vi "RGBtoGray.vi"() -> ()   [LabVIEW 2019]
uses:
  <vilib>/vision/NI_Vision_Development_Module.lvlib
  RGB_To_Gray DLL Project/Project RGBToGray VI/RGBToGray.dll
panel:
  out "Gray Image Built In function":T1(plugin-control)
  out "Gray Image":T1(plugin-control)
  out "Execution Time in seconds (in DLL)":dbl
  out "Original Image":T1(plugin-control)
  in  "File Path":path
  out "Elapsed Time Labview Built in VI in ms":u32
  out "Elapsed Time For Our C DLL in ms":u32
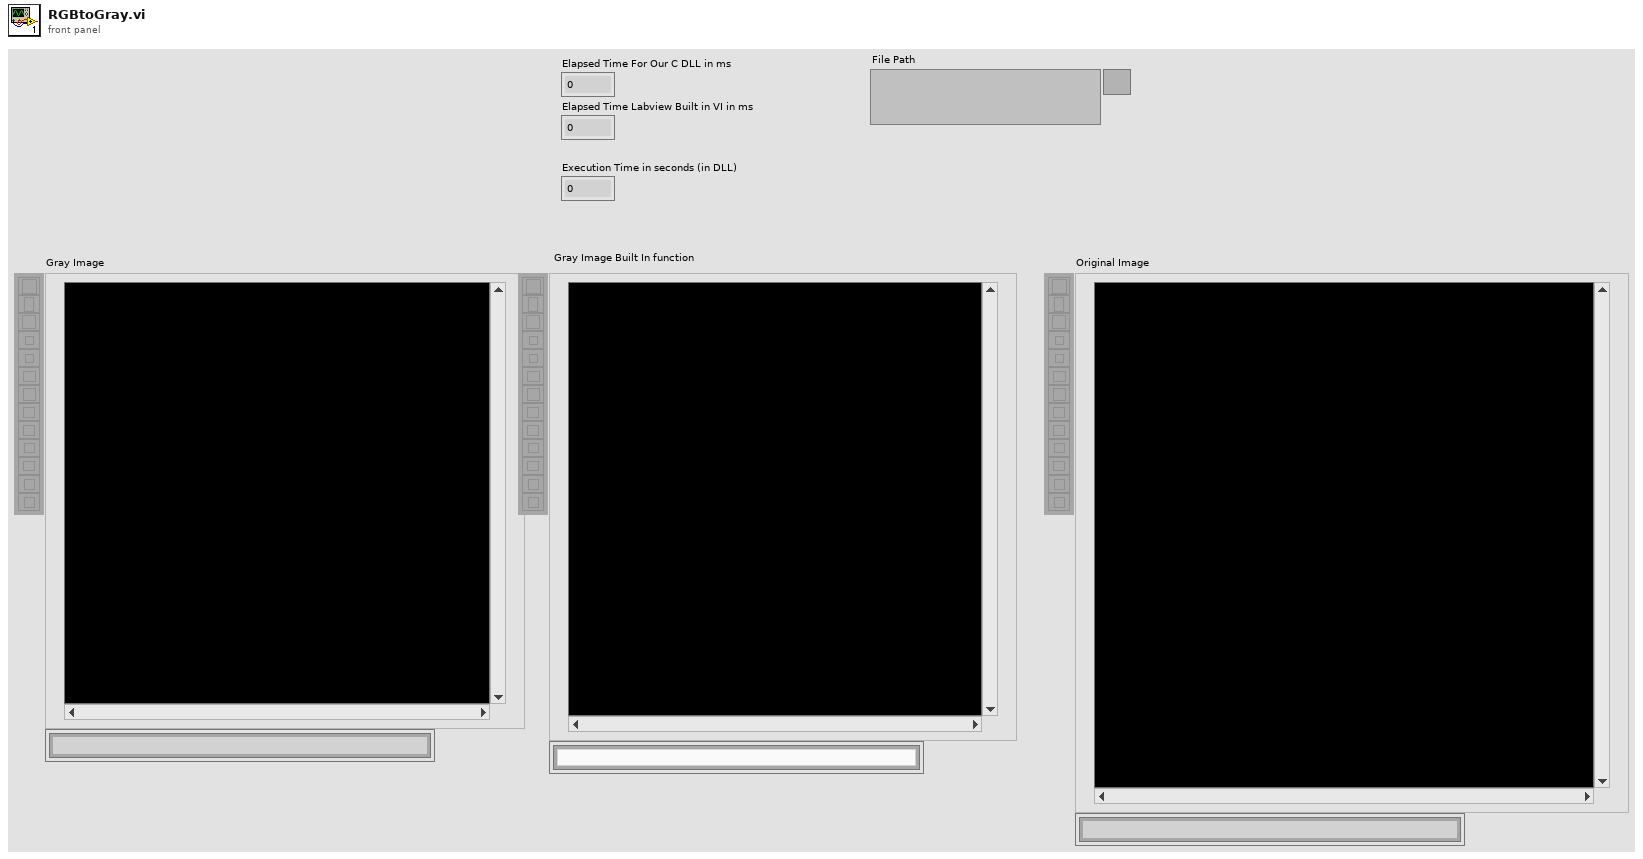
[diagram p1: front panel]
types:
  T1 = typedef "IMAQ Image.ctl" = refnum<image>
  T2 = enum32{"Map Pixel Pointer", "Unmap Pixel Pointer", "Get Pixels Infos"}
  T3 = typedef "Image Type" = u32
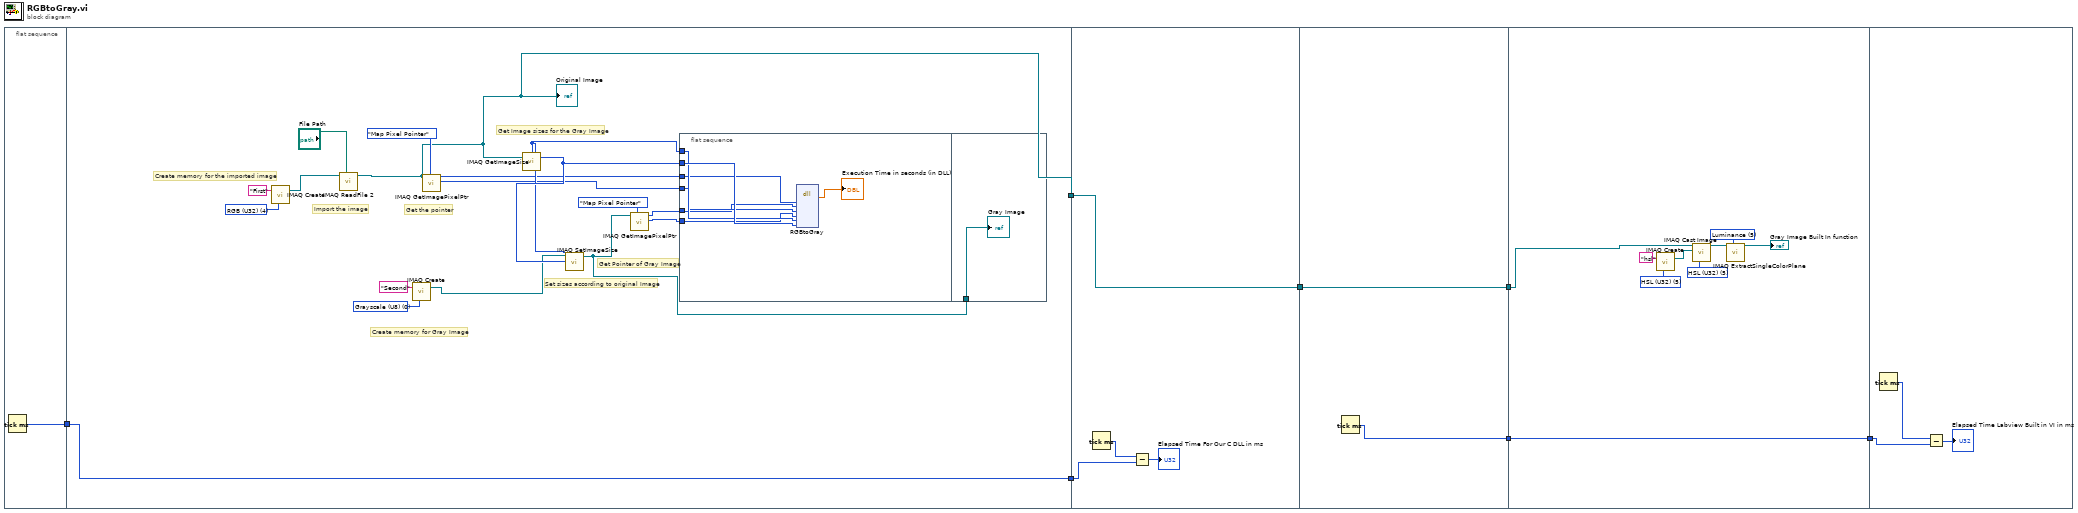
[diagram p0: block diagram]
diagram:
  n1 = flat-sequence {
    tunnel: [w8] -> w7
    tunnel: w7 -> [w26]
    tunnel: [w26] -> w6
    tunnel: [w11] -> w5
    tunnel: w6 -> [w37]
    tunnel: [w35] -> w4
    tunnel: w5 -> [w35]
    tunnel: [w40] -> w3
    tunnel: w4 -> [w39]
    tunnel: [w39] -> w2
    tunnel: w3 -> [w49]
    tunnel: [w49] -> w1
    tunnel: w2 -> [w42]
    tunnel: w1 -> [w52]
    frame #0 {
      n2 = Tick Count (ms)() -> (millisecond timer value=w8:u32)
    }
    frame #1 {
      w19 = T3 0 items=["Grayscale (U8)", "Grayscale (I16)", "Grayscale (SGL)", "Complex (CSG)", "RGB (U32)", "HSL (U32)", "RGB (U64)", "Grayscale (U16)"] ("Image Type")
      w23 = T3 4 items=["Grayscale (U8)", "Grayscale (I16)", "Grayscale (SGL)", "Complex (CSG)", "RGB (U32)", "HSL (U32)", "RGB (U64)", "Grayscale (U16)"] ("Image Type")
      # "Get Pointer of Gray Image"
      # "Set sizes according to original Image"
      # "Create memory for Gray Image"
      # "Get Image sizes for the Gray Image"
      # "Get the pointer"
      # "Import the image"
      # "Create memory for the imported image"
      n3 = call "IMAQ Create"("Image Name"="First", "Image Type"=w23) -> ("New Image"=w22:T1)  [unwired: 3 in, 1 out]
      n4 = call "IMAQ ReadFile 2"("File Path"="File Path", "Image"=w22) -> ("Image Out"=w11:T1)  [unwired: 5 in, 4 out]
      "Original Image" <- w11
      n5 = call "IMAQ Create"("Image Name"="Second", "Image Type"=w19) -> ("New Image"=w10:T1)  [unwired: 3 in, 1 out]
      n6 = call "IMAQ GetImagePixelPtr"("Function"=T2."Map Pixel Pointer", "Image"=w11) -> ("LineWidth(Pixels)"=w13:i32, "Pixel Pointer out"=w14:u64)  [unwired: 4 in, 4 out]
      n7 = call "IMAQ GetImageSize"("Image"=w11) -> ("Y Resolution"=w17:i32, "X Resolution"=w15:i32)  [unwired: 3 in, 1 out]
      n8 = call "IMAQ SetImageSize"("Y Resolution"=w17, "X Resolution"=w15, "Image"=w10) -> ("Image Out"=w9:T1)  [unwired: 2 in, 1 out]
      n9 = call "IMAQ GetImagePixelPtr"("Function"=T2."Map Pixel Pointer", "Image"=w9) -> ("LineWidth(Pixels)"=w12:i32, "Pixel Pointer out"=w16:u64)  [unwired: 4 in, 4 out]
      n10 = flat-sequence {
        tunnel: w17 -> [w33]
        tunnel: w15 -> [w32]
        tunnel: w16 -> [w29]
        tunnel: w14 -> [w28]
        tunnel: w13 -> [w30]
        tunnel: w12 -> [w31]
        tunnel: w9 -> [w34]
        frame #0 {
          n11 = dll-call lib="C:/Users/byald/Desktop/EE-433 Project Group1/RGB_To_Gray DLL Project/Project RGBToGray VI/RGBToGray.dll" fn="RGBtoGray"("RGBImage"=w28, "GrayImage"=w29, "LVLineWidthRGB"=w30, "LVLineWidthGray"=w31, "LVWidth"=w32, "LVHeight"=w33) -> ("return type"=→"Execution Time in seconds (in DLL)":dbl)  [unwired: 9 in, 2 out]
        }
        frame #1 {
          "Gray Image" <- w34
        }
      }
    }
    frame #2 {
      n12 = Tick Count (ms)() -> (millisecond timer value=w38:u32)
      n13 = Subtract(x=w38, y=w37) -> (x-y=→"Elapsed Time For Our C DLL in ms":u32)
    }
    frame #3 {
      n14 = Tick Count (ms)() -> (millisecond timer value=w40:u32)
    }
    frame #4 {
      w43 = 5 items=["Red", "Green", "Blue", "Hue", "Saturation", "Luminance", "Value", "Intensity"] ("Color Plane")
      w45 = T3 5 items=["Grayscale (U8)", "Grayscale (I16)", "Grayscale (SGL)", "Complex (CSG)", "RGB (U32)", "HSL (U32)", "RGB (U64)"] ("Image Type")
      w46 = T3 5 items=["Grayscale (U8)", "Grayscale (I16)", "Grayscale (SGL)", "Complex (CSG)", "RGB (U32)", "HSL (U32)", "RGB (U64)"] ("Image Type")
      n15 = call "IMAQ Create"("Image Name"="hsl", "Image Type"=w46) -> ("New Image"=w48:T1)  [unwired: 2 in, 2 out]
      n16 = call "IMAQ Cast Image"("Image Type"=w45, "Image Dst"=w48, "Image Src"=w42) -> ("Image Dst Out"=w44:T1)  [unwired: 3 in, 5 out]
      n17 = call "IMAQ ExtractSingleColorPlane"("Color Plane"=w43, "Image Src"=w44) -> ("Image Dst Out"=→"Gray Image Built In function":T1)  [unwired: 2 in, 7 out]
    }
    frame #5 {
      n18 = Tick Count (ms)() -> (millisecond timer value=w51:u32)
      n19 = Subtract(x=w51, y=w52) -> (x-y=→"Elapsed Time Labview Built in VI in ms":u32)
    }
  }
